vi "sub vi - calibration v2.vi"(6 "Samples":dbl, 8 "Task2":dbl, 9 "Task1":dbl, 10 "Task0":dbl, 11 "Temp Test Cal":dbl) -> ()   [LabVIEW 2017]
panel:
  out "UPDATE":bool
  in  "stop":bool
  in  "Tab Control":T1(tab)
  out "1-2(TN) Run":dbl
  out "1-2(TL) Run":dbl
  out "1-1(TN) Run":dbl
  out "1-1(TL) Run":dbl
  out "LAB01-1 (GRAPH)":dynamicdata(graph)
  out "LAB01-2 (GRAPH)":dynamicdata(graph)
  in  "LAB01 (CAL)":T2 {"2 (TN) cal" min=0.0 step=0.01 format="%.2f"; "2 (TL) cal" min=0.0 step=0.01 format="%.2f"; "2 (PF) cal" min=0.0 step=0.01 format="%.2f"; "2 (V) cal" min=0.0 step=0.01 format="%.2f"; "2 (A) cal" min=0.0 step=0.01 format="%.2f"; "1 (TN) cal" min=0.0 step=0.01 format="%.2f"; "1 (TL) cal" min=0.0 step=0.01 format="%.2f"; "1 (PF) cal" min=0.0 step=0.01 format="%.2f"; "1 (V) cal" min=0.0 step=0.01 format="%.2f"; "1  (A) cal" min=0.0 step=0.01 format="%.2f"}
  out "LAB01 (SIGNALS)":T3 {"2 (PF)" format="%.2f"; "2 (A)" format="%.1f"; "1 (PF)" format="%.2f"; "1 (A)" format="%.1f"}
  out "2-2(TN) Run":dbl
  out "2-2(TL) Run":dbl
  out "2-1(TN) Run":dbl
  out "2-1(TL) Run":dbl
  out "LAB02 (SIGNALS)":T3 {"2 (PF)" format="%.2f"; "2 (A)" format="%.1f"; "1 (PF)" format="%.2f"; "1 (A)" format="%.1f"}
  in  "LAB02 (CAL)":T4 {"2 (TN) cal" min=0.0 step=0.01 format="%.2f"; "2 (TL) cal" min=0.0 step=0.01 format="%.2f"; "2 (PF) cal" min=0.0 step=0.01 format="%.2f"; "2 (V) cal" min=0.0 step=0.01 format="%.2f"; "2 (A) cal" min=0.0 step=0.01 format="%.2f"; "1 (TN) cal" min=0.0 step=0.01 format="%.2f"; "1 (TL) cal" min=0.0 step=0.01 format="%.2f"; "1 (PF) cal" min=0.0 step=0.01 format="%.2f"; "1 (V) cal" min=0.0 step=0.01 format="%.2f"; "1 (A) cal" min=0.0 step=0.01 format="%.2f"}
  out "LAB02-2 (GRAPH)":dynamicdata(graph)
  out "LAB02-1 (GRAPH)":dynamicdata(graph)
  out "3-2(TN) Run":dbl
  out "3-2(TL) Run":dbl
  out "3-1(TN) Run":dbl
  out "3-1(TL) Run":dbl
  out "LAB03 (SIGNALS)":T3 {"2 (PF)" format="%.2f"; "2 (A)" format="%.1f"; "1 (PF)" format="%.2f"; "1 (A)" format="%.1f"}
  in  "LAB03 (CAL)":T2 {"2 (TN) cal" min=0.0 step=0.01 format="%.2f"; "2 (TL) cal" min=0.0 step=0.01 format="%.2f"; "2 (PF) cal" min=0.0 step=0.01 format="%.2f"; "2 (V) cal" min=0.0 step=0.01 format="%.2f"; "2 (A) cal" min=0.0 step=0.01 format="%.2f"; "1 (TN) cal" min=0.0 step=0.01 format="%.2f"; "1 (TL) cal" min=0.0 step=0.01 format="%.2f"; "1 (PF) cal" min=0.0 step=0.01 format="%.2f"; "1 (V) cal" min=0.0 step=0.01 format="%.2f"; "1  (A) cal" min=0.0 step=0.01 format="%.2f"}
  out "LAB03-2 (GRAPH)":dynamicdata(graph)
  out "LAB03-1 (GRAPH)":dynamicdata(graph)
  out "4-2(TN) Run":dbl
  out "4-2(TL) Run":dbl
  out "4-1(TN) Run":dbl
  out "4-1(TL) Run":dbl
  out "LAB04 (SIGNALS)":T3 {"2 (PF)" format="%.2f"; "2 (A)" format="%.1f"; "1 (PF)" format="%.2f"; "1 (A)" format="%.1f"}
  in  "LAB04 (CAL)":T2 {"2 (TN) cal" min=0.0 step=0.01 format="%.2f"; "2 (TL) cal" min=0.0 step=0.01 format="%.2f"; "2 (PF) cal" min=0.0 step=0.01 format="%.2f"; "2 (V) cal" min=0.0 step=0.01 format="%.2f"; "2 (A) cal" min=0.0 step=0.01 format="%.2f"; "1 (TN) cal" min=0.0 step=0.01 format="%.2f"; "1 (TL) cal" min=0.0 step=0.01 format="%.2f"; "1 (PF) cal" min=0.0 step=0.01 format="%.2f"; "1 (V) cal" min=0.0 step=0.01 format="%.2f"; "1  (A) cal" min=0.0 step=0.01 format="%.2f"}
  out "LAB04-2 (GRAPH)":dynamicdata(graph)
  out "LAB04-1 (GRAPH)":dynamicdata(graph)
  in  "LAB05 (CAL) 2":T5 {"2  (A)Zero Offset 1" min=0.0 step=0.01 format="%.2f"; "1  (A)Zero Offset" min=0.0 step=0.01 format="%.2f"; "2 (TN) cal" min=0.0 step=0.01 format="%.2f"; "2 (TL) cal" min=0.0 step=0.01 format="%.2f"; "2 (PF) cal" min=0.0 step=0.01 format="%.2f"; "2 (V) cal" min=0.0 step=0.01 format="%.2f"; "2 (A) cal" min=0.0 step=0.01 format="%.2f"; "1 (TN) cal" min=0.0 step=0.01 format="%.2f"; "1 (TL) cal" min=0.0 step=0.01 format="%.2f"; "1 (PF) cal" min=0.0 step=0.01 format="%.2f"; "1 (V) cal" min=0.0 step=0.01 format="%.2f"; "1  (A) cal" min=0.0 step=0.01 format="%.2f"}
  out "5-2(TN) Run":dbl
  out "5-2(TL) Run":dbl
  out "5-1(TN) Run":dbl
  out "5-1(TL) Run":dbl
  out "LAB05 (SIGNALS)":T3 {"2 (PF)" format="%.2f"; "2 (A)" format="%.1f"; "1 (PF)" format="%.2f"; "1 (A)" format="%.1f"}
  out "LAB05-2 (GRAPH)":dynamicdata(graph)
  out "LAB05-1 (GRAPH)":dynamicdata(graph)
  in  "TEMP REF cal":dbl
  out "AMBIENT TEMP REF":dbl format="%.1f"
  out "Data2":waveform(dbl)[](graph)
  out "Data1":waveform(dbl)[](graph)
  out "Data0":waveform(dbl)[](graph)
  out "Analog Loop Time":dbl
  out "Temperature data error":bool
  out "file error out":errorcluster
  out "AI Error":errorcluster[](array[cluster])
  out "data 0":waveform(dbl)[](array[waveform])
  out "data 1":waveform(dbl)[](array[waveform])
  out "data 2":waveform(dbl)[](array[waveform])
  # "This value is only applied during\ntesting to adjust for insulatred probe\nprofile during current flow temp rise.\nIf any change is made here, make sure\nvalue is changed to same value on\nADM tab."
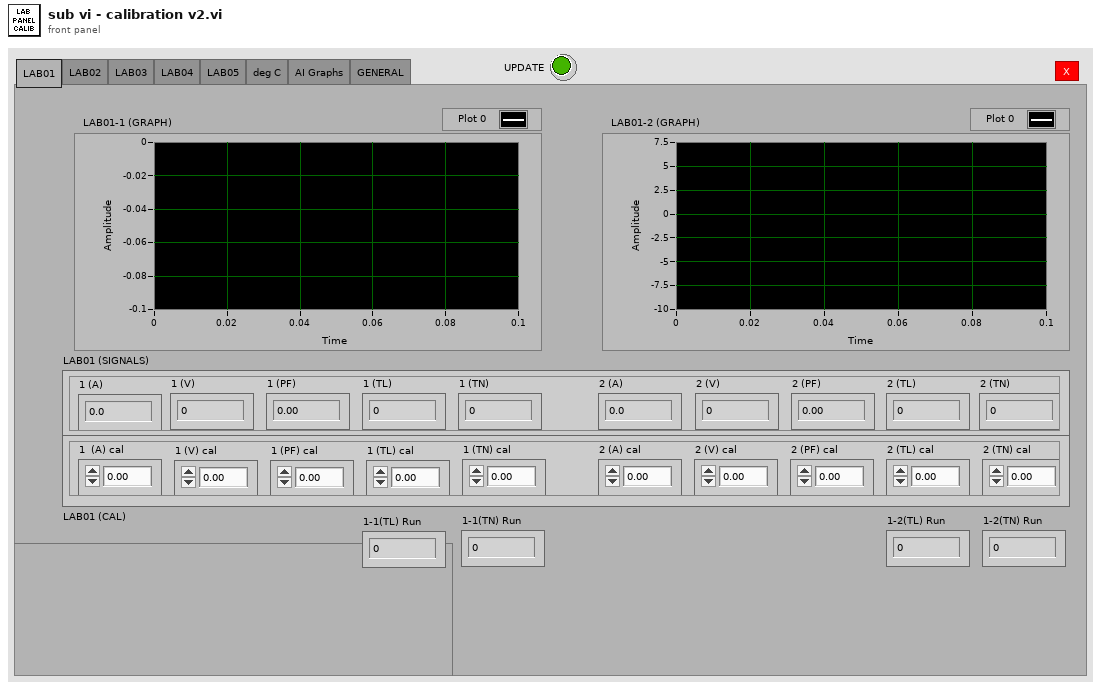
[diagram p1: front panel]
types:
  T1 = enum32{"LAB01", "LAB02", "LAB03", "LAB04", "LAB05", "deg C", "AI Graphs", "GENERAL"}
  T2 = cluster{"1  (A) cal":dbl, "1 (V) cal":dbl, "1 (PF) cal":dbl, "1 (TL) cal":dbl, "1 (TN) cal":dbl, "2 (A) cal":dbl, "2 (V) cal":dbl, "2 (PF) cal":dbl, "2 (TL) cal":dbl, "2 (TN) cal":dbl}
  T3 = cluster{"1 (TL)":dbl, "1 (TN)":dbl, "2 (TL)":dbl, "2 (TN)":dbl, "1 (A)":dbl, "1 (V)":dbl, "1 (PF)":dbl, "2 (A)":dbl, "2 (V)":dbl, "2 (PF)":dbl}
  T4 = cluster{"1 (A) cal":dbl, "1 (V) cal":dbl, "1 (PF) cal":dbl, "1 (TL) cal":dbl, "1 (TN) cal":dbl, "2 (A) cal":dbl, "2 (V) cal":dbl, "2 (PF) cal":dbl, "2 (TL) cal":dbl, "2 (TN) cal":dbl}
  T5 = cluster{"1  (A) cal":dbl, "1 (V) cal":dbl, "1 (PF) cal":dbl, "1 (TL) cal":dbl, "1 (TN) cal":dbl, "2 (A) cal":dbl, "2 (V) cal":dbl, "2 (PF) cal":dbl, "2 (TL) cal":dbl, "2 (TN) cal":dbl, "1  (A)Zero Offset":dbl, "2  (A)Zero Offset 1":dbl}
  T6 = enum16{"open", "replace", "create", "open or create", "replace or create", "replace or create with confirmation"}
  T7 = cluster{"LAB01-1 (A)":dbl, "LAB01-1 (V)":dbl, "LAB01-1 (PF)":dbl, "LAB01-2 (A)":dbl, "LAB01-2 (V)":dbl, "LAB01-2 (PF)":dbl}
  T8 = cluster{"LAB02-1 (A)":dbl, "LAB02-1 (V)":dbl, "LAB02-1 (PF)":dbl, "LAB02-2 (A)":dbl, "LAB02-2 (V)":dbl, "LAB02-2 (PF)":dbl}
  T9 = cluster{"LAB03-1 (A)":dbl, "LAB03-1 (V)":dbl, "LAB03-1 (PF)":dbl, "LAB03-2 (A)":dbl, "LAB03-2 (V)":dbl, "LAB03-2 (PF)":dbl}
  T10 = cluster{"LAB04-1 (A)":dbl, "LAB04-1 (V)":dbl, "LAB04-1 (PF)":dbl, "LAB04-2 (A)":dbl, "LAB04-2 (V)":dbl, "LAB04-2 (PF)":dbl}
  T11 = cluster{"LAB05-1 (A)":dbl, "LAB05-1 (V)":dbl, "LAB05-1 (PF)":dbl, "LAB05-2 (A)":dbl, "LAB05-2 (V)":dbl, "LAB05-2 (PF)":dbl}
  T12 = cluster{"T1":dbl, "T2":dbl, "T3":dbl, "T4":dbl, "ID":dbl, "ER":dbl}
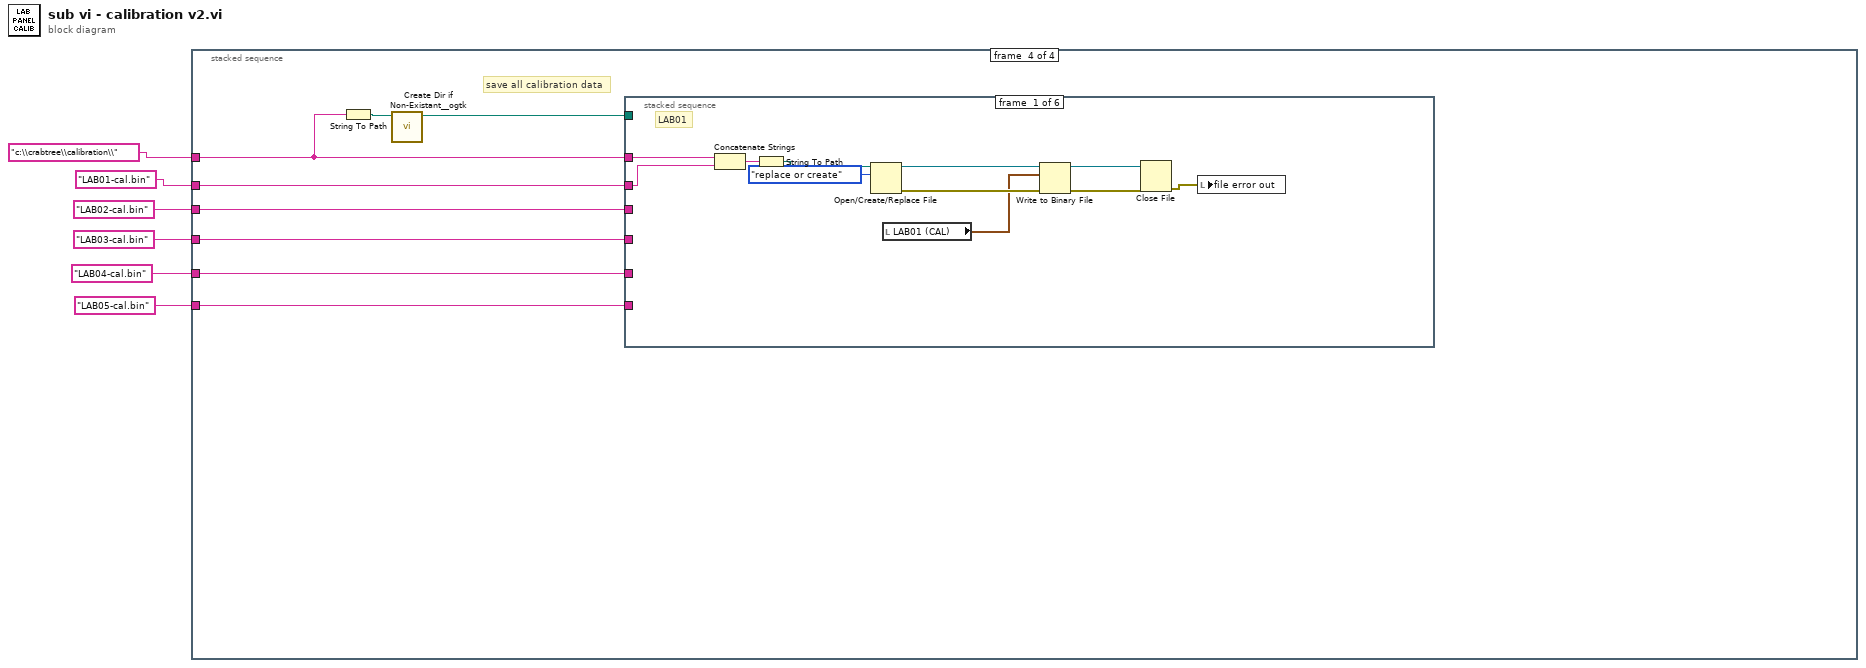
[diagram p0: block diagram]
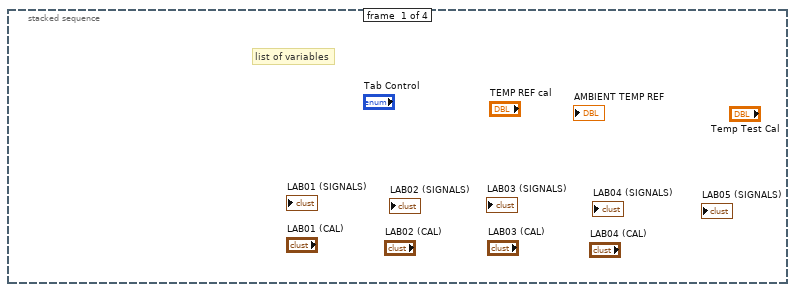
[diagram p2: hidden frame]
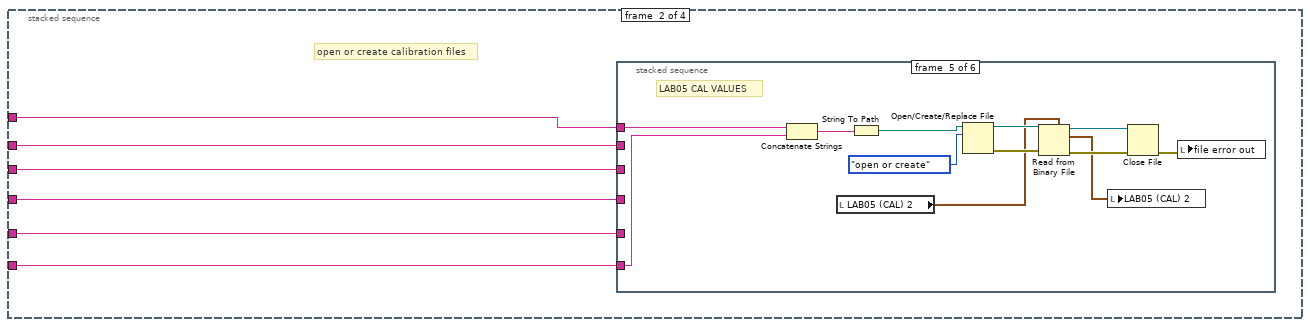
[diagram p3: hidden frame]
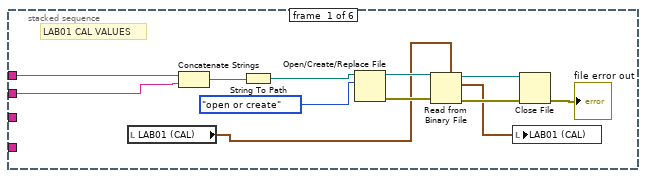
[diagram p4: hidden frame]
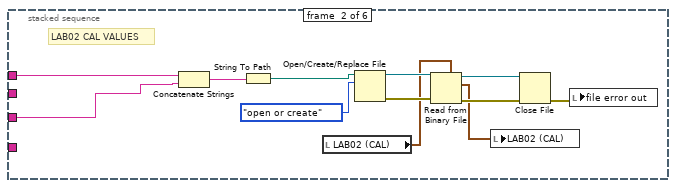
[diagram p5: hidden frame]
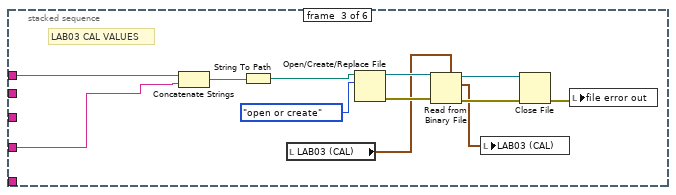
[diagram p6: hidden frame]
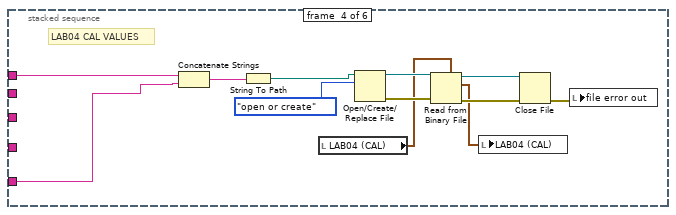
[diagram p7: hidden frame]
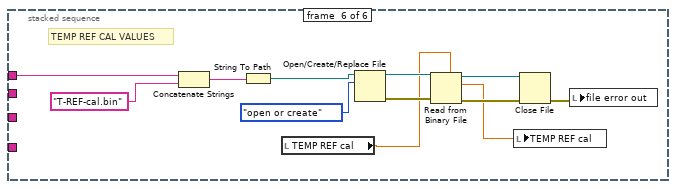
[diagram p8: hidden frame]
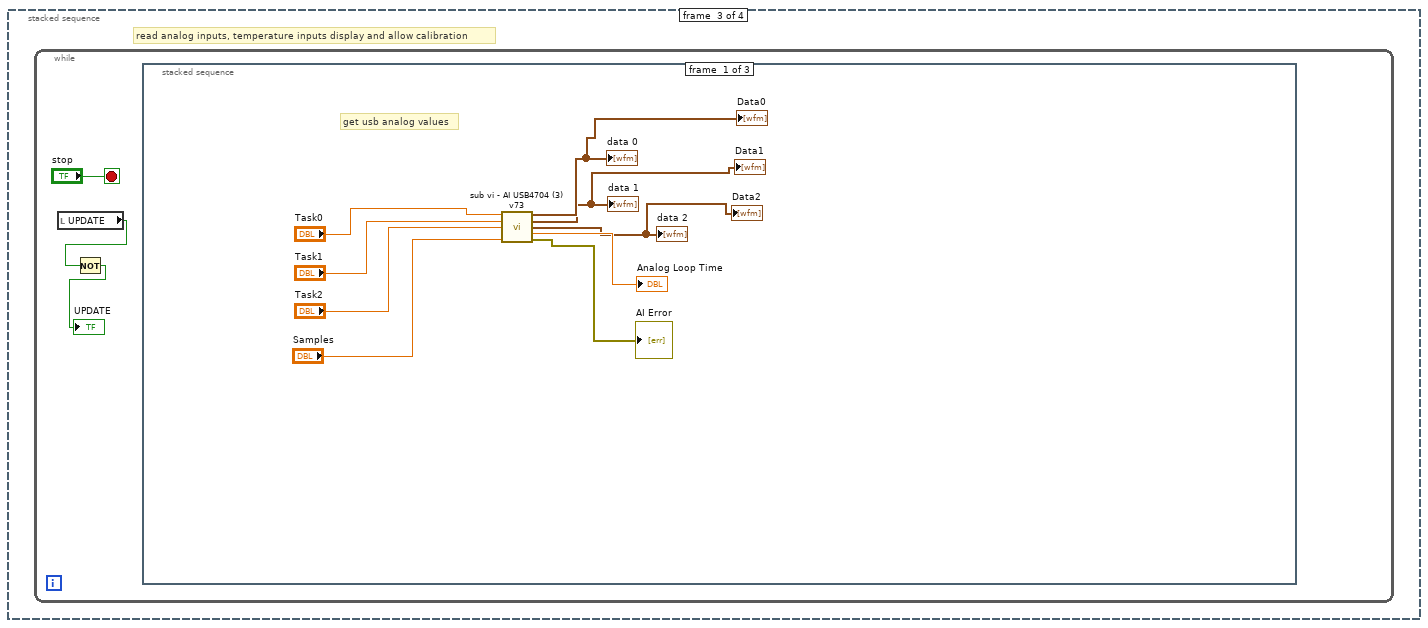
[diagram p9: hidden frame]
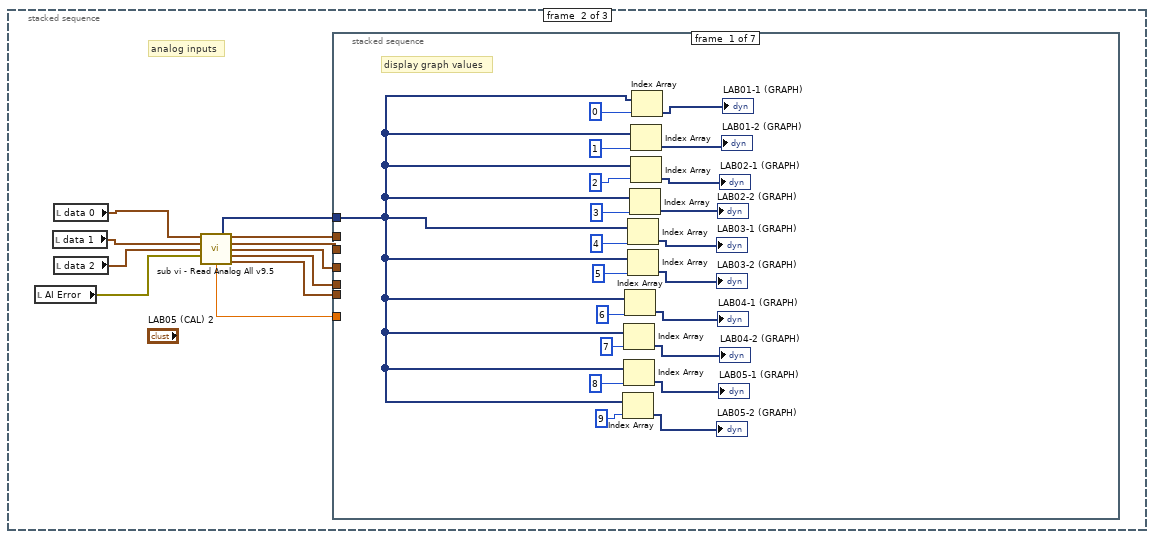
[diagram p10: hidden frame]
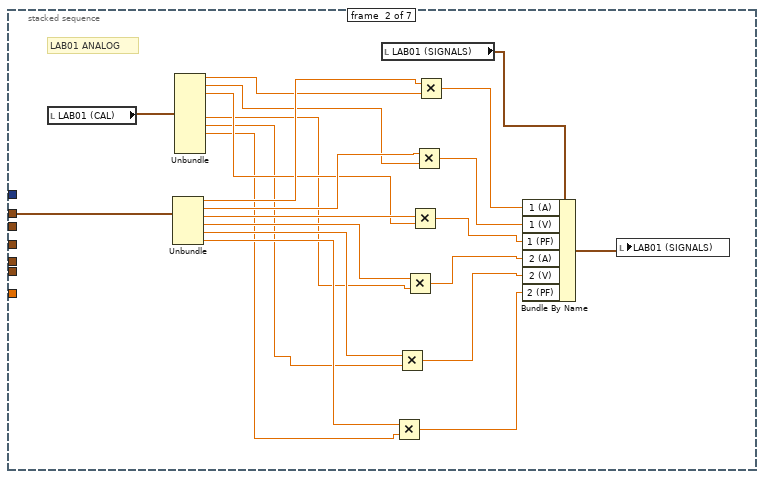
[diagram p11: hidden frame]
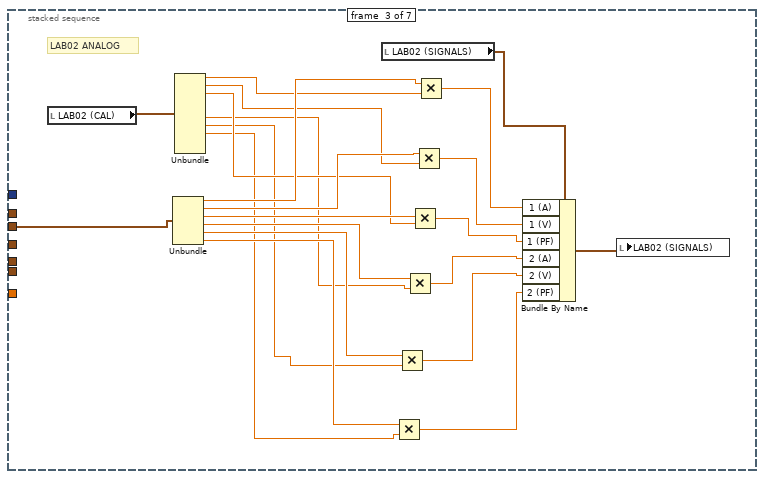
[diagram p12: hidden frame]
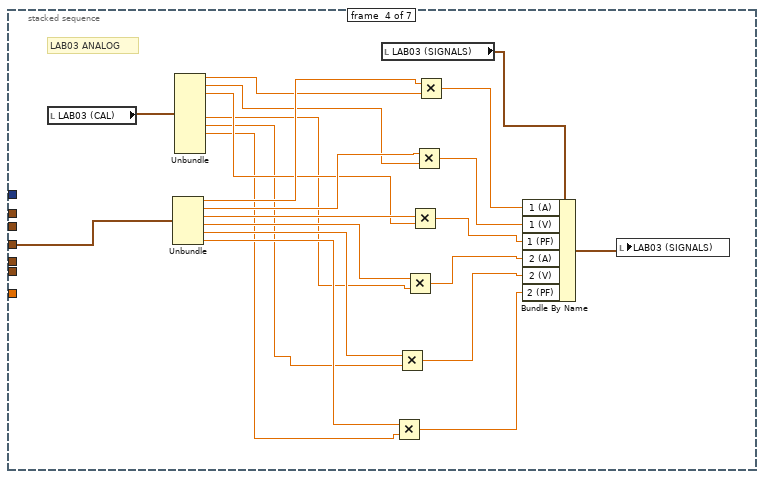
[diagram p13: hidden frame]
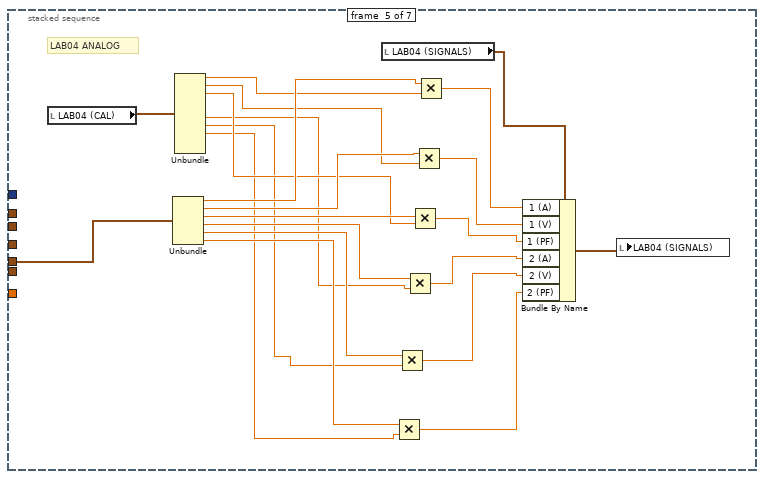
[diagram p14: hidden frame]
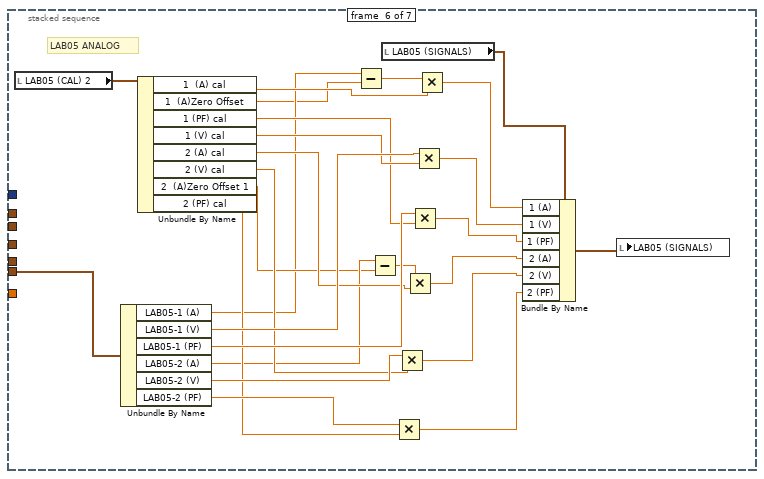
[diagram p15: hidden frame]
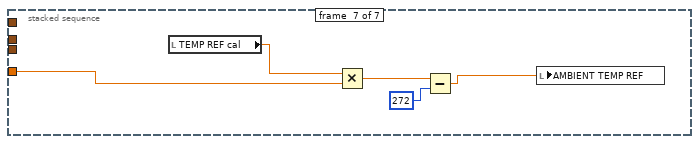
[diagram p16: hidden frame]
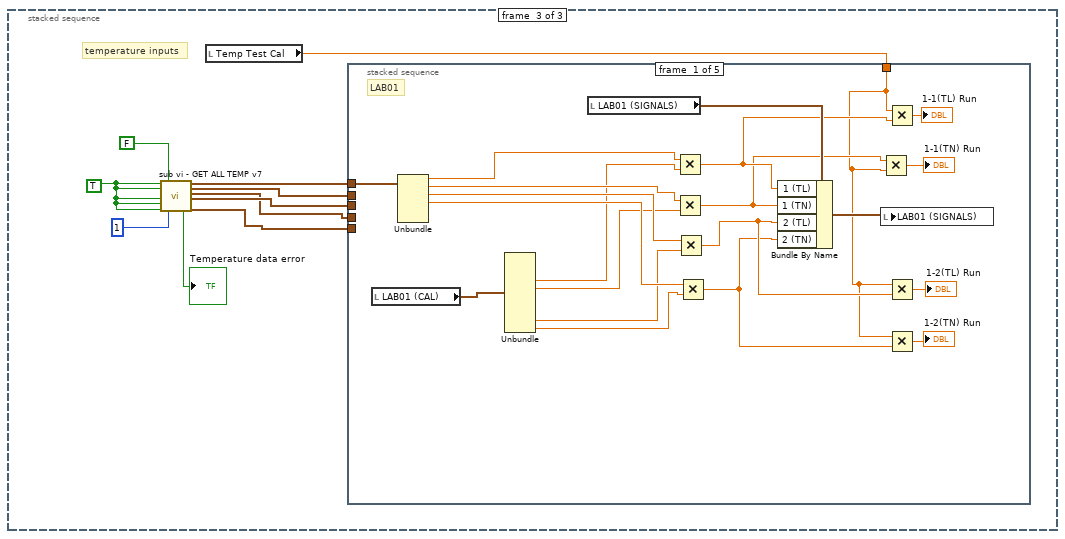
[diagram p17: hidden frame]
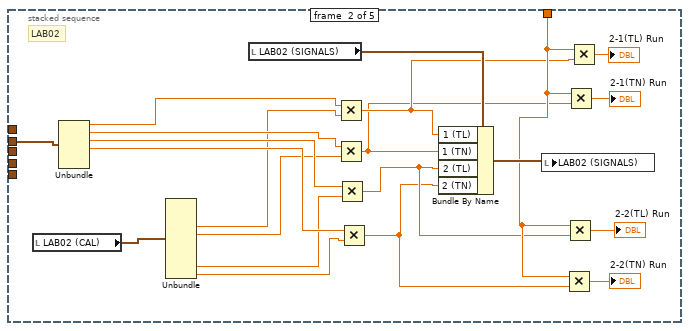
[diagram p18: hidden frame]
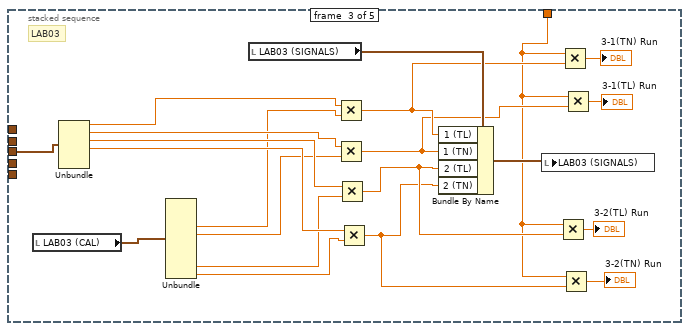
[diagram p19: hidden frame]
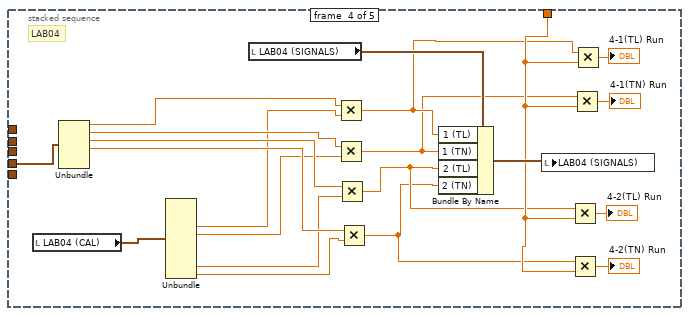
[diagram p20: hidden frame]
diagram:
  n1 = stacked-sequence {
    tunnel: "c:\\crabtree\\calibration\\" -> [_ w12 _ w365]
    tunnel: "LAB01-cal.bin" -> [_ w11 _ w370]
    tunnel: "LAB02-cal.bin" -> [_ w10 _ w369]
    tunnel: "LAB03-cal.bin" -> [_ w9 _ w368]
    tunnel: "LAB04-cal.bin" -> [_ w8 _ w367]
    tunnel: "LAB05-cal.bin" -> [_ w7 _ w366]
    frame #0 {
      # "list of variables"
    }
    frame #1 {
      # "open or create calibration files"
      n2 = stacked-sequence {
        tunnel: w12 -> [w24 w36 w48 w60 w72 w84]
        tunnel: w11 -> [w15 _ _ _ _ _]
        tunnel: w10 -> [_ w27 _ _ _ _]
        tunnel: w9 -> [_ _ w39 _ _ _]
        tunnel: w8 -> [_ _ _ w52 _ _]
        tunnel: w7 -> [_ _ _ _ w63 _]
        frame #0 {
          # "LAB01 CAL VALUES"
          n3 = local read "LAB01 (CAL)"() -> (w14:T2)
          n4 = Concatenate Strings(w24, w15) -> (w23:string)
          n5 = String To Path(string=w23) -> (path=w22:path)
          n6 = Open/Create/Replace File(file path (use dialog)=w22, operation (0:open)=T6."open or create") -> (refnum out=w21:refnum<file>, error out=w20:errorcluster)  [unwired: 4 in, 1 out]
          n7 = Read from Binary File(5:w14, 8:w20, 11:w21) -> (0:w18:errorcluster, 2:w13:T2, 3:w19:refnum<file>)  [unwired: 3 in, 1 out]
          n8 = local write "LAB01 (CAL)"(w13) -> ()
          n9 = Close File(refnum=w19, error in=w18) -> (error out=→"file error out":errorcluster)  [unwired: 1 out]
        }
        frame #1 {
          # "LAB02 CAL VALUES"
          n10 = Concatenate Strings(w36, w27) -> (w35:string)
          n11 = String To Path(string=w35) -> (path=w34:path)
          n12 = local read "LAB02 (CAL)"() -> (w26:T4)
          n13 = Open/Create/Replace File(file path (use dialog)=w34, operation (0:open)=T6."open or create") -> (refnum out=w33:refnum<file>, error out=w32:errorcluster)  [unwired: 4 in, 1 out]
          n14 = Read from Binary File(5:w26, 8:w32, 11:w33) -> (0:w30:errorcluster, 2:w25:T4, 3:w31:refnum<file>)  [unwired: 3 in, 1 out]
          n15 = local write "LAB02 (CAL)"(w25) -> ()
          n16 = Close File(refnum=w31, error in=w30) -> (error out=w28:errorcluster)  [unwired: 1 out]
          n17 = local write "file error out"(w28) -> ()
        }
        frame #2 {
          # "LAB03 CAL VALUES"
          n18 = Concatenate Strings(w48, w39) -> (w47:string)
          n19 = String To Path(string=w47) -> (path=w46:path)
          n20 = local read "LAB03 (CAL)"() -> (w38:T2)
          n21 = Open/Create/Replace File(file path (use dialog)=w46, operation (0:open)=T6."open or create") -> (refnum out=w45:refnum<file>, error out=w44:errorcluster)  [unwired: 4 in, 1 out]
          n22 = Read from Binary File(5:w38, 8:w44, 11:w45) -> (0:w42:errorcluster, 2:w37:T2, 3:w43:refnum<file>)  [unwired: 3 in, 1 out]
          n23 = local write "LAB03 (CAL)"(w37) -> ()
          n24 = Close File(refnum=w43, error in=w42) -> (error out=w40:errorcluster)  [unwired: 1 out]
          n25 = local write "file error out"(w40) -> ()
        }
        frame #3 {
          # "LAB04 CAL VALUES"
          n26 = Concatenate Strings(w60, w52) -> (w59:string)
          n27 = String To Path(string=w59) -> (path=w58:path)
          n28 = local read "LAB04 (CAL)"() -> (w50:T2)
          n29 = Open/Create/Replace File(file path (use dialog)=w58, operation (0:open)=T6."open or create") -> (refnum out=w57:refnum<file>, error out=w56:errorcluster)  [unwired: 4 in, 1 out]
          n30 = Read from Binary File(5:w50, 8:w56, 11:w57) -> (0:w54:errorcluster, 2:w49:T2, 3:w55:refnum<file>)  [unwired: 3 in, 1 out]
          n31 = local write "LAB04 (CAL)"(w49) -> ()
          n32 = Close File(refnum=w55, error in=w54) -> (error out=w53:errorcluster)  [unwired: 1 out]
          n33 = local write "file error out"(w53) -> ()
        }
        frame #4 {
          # "LAB05 CAL VALUES"
          n34 = Concatenate Strings(w72, w63) -> (w71:string)
          n35 = local read "LAB05 (CAL) 2"() -> (w62:T5)
          n36 = String To Path(string=w71) -> (path=w70:path)
          n37 = Open/Create/Replace File(file path (use dialog)=w70, operation (0:open)=T6."open or create") -> (refnum out=w69:refnum<file>, error out=w68:errorcluster)  [unwired: 4 in, 1 out]
          n38 = Read from Binary File(5:w62, 8:w68, 11:w69) -> (0:w66:errorcluster, 2:w61:T5, 3:w67:refnum<file>)  [unwired: 3 in, 1 out]
          n39 = local write "LAB05 (CAL) 2"(w61) -> ()
          n40 = Close File(refnum=w67, error in=w66) -> (error out=w64:errorcluster)  [unwired: 1 out]
          n41 = local write "file error out"(w64) -> ()
        }
        frame #5 {
          # "TEMP REF CAL VALUES"
          n42 = Concatenate Strings(w84, "T-REF-cal.bin") -> (w83:string)
          n43 = String To Path(string=w83) -> (path=w82:path)
          n44 = local read "TEMP REF cal"() -> (w74:dbl)
          n45 = Open/Create/Replace File(file path (use dialog)=w82, operation (0:open)=T6."open or create") -> (refnum out=w81:refnum<file>, error out=w80:errorcluster)  [unwired: 4 in, 1 out]
          n46 = Read from Binary File(5:w74, 8:w80, 11:w81) -> (0:w78:errorcluster, 2:w73:dbl, 3:w79:refnum<file>)  [unwired: 3 in, 1 out]
          n47 = local write "TEMP REF cal"(w73) -> ()
          n48 = Close File(refnum=w79, error in=w78) -> (error out=w76:errorcluster)  [unwired: 1 out]
          n49 = local write "file error out"(w76) -> ()
        }
      }
    }
    frame #2 {
      # "read analog inputs, temperature inputs display and allow calibration"
      n50 = while {
        stop <- "stop" stop-if-true
        n51 = local read "UPDATE"() -> (w85:bool)
        n52 = Not(x=w85) -> (.not. x?=→"UPDATE":bool)
        n53 = stacked-sequence {
          frame #0 {
            # "get usb analog values"
            n54 = call "sub vi - AI USB4704 (3) v73.vi"("Task0"="Task0", "Task1"="Task1", "Task2"="Task2", "SAMPLES"="Samples") -> ("data 0"=→"data 0" →"Data0":waveform(dbl)[], "data 1"=→"data 1" →"Data1":waveform(dbl)[], "data 2"=→"data 2" →"Data2":waveform(dbl)[], "loop time"=→"Analog Loop Time":dbl, "error array"=→"AI Error":errorcluster[])  [unwired: 5 in, 2 out]
          }
          frame #1 {
            # "analog inputs"
            n55 = local read "AI Error"() -> (w97:errorcluster[])
            n56 = local read "data 1"() -> (w99:waveform(dbl)[])
            n57 = local read "data 0"() -> (w100:waveform(dbl)[])
            n58 = local read "data 2"() -> (w98:waveform(dbl)[])
            n59 = call "sub vi - Read Analog All v9.5.vi"("data 0"=w100, "data 1"=w99, "data 2"=w98, "AI Error"=w97) -> ("array GRAPH"=w107:dynamicdata[], "LAB01"=w106:T7, "LAB02"=w105:T8, "LAB03"=w104:T9, "LAB04"=w103:T10, "deg C"=w101:dbl, "LAB05"=w102:T11)  [unwired: 3 in, 2 out]
            n60 = stacked-sequence {
              tunnel: w107 -> [w127 _ _ _ _ _ _]
              tunnel: w106 -> [_ w149 _ _ _ _ _]
              tunnel: w104 -> [_ _ _ w173 _ _ _]
              tunnel: w105 -> [_ _ w151 _ _ _ _]
              tunnel: w103 -> [_ _ _ _ w195 _ _]
              tunnel: w102 -> [_ _ _ _ _ w228 _]
              tunnel: w101 -> [_ _ _ _ _ _ w246]
              frame #0 {
                # "display graph values"
                n61 = Index Array(array=w127, index=9) -> (element=→"LAB05-2 (GRAPH)":dynamicdata)
                n62 = Index Array(array=w127, index=7) -> (element=→"LAB04-2 (GRAPH)":dynamicdata)
                n63 = Index Array(array=w127, index=8) -> (element=→"LAB05-1 (GRAPH)":dynamicdata)
                n64 = Index Array(array=w127, index=6) -> (element=→"LAB04-1 (GRAPH)":dynamicdata)
                n65 = Index Array(array=w127, index=4) -> (element=→"LAB03-1 (GRAPH)":dynamicdata)
                n66 = Index Array(array=w127, index=5) -> (element=→"LAB03-2 (GRAPH)":dynamicdata)
                n67 = Index Array(array=w127, index=3) -> (element=→"LAB02-2 (GRAPH)":dynamicdata)
                n68 = Index Array(array=w127, index=1) -> (element=→"LAB01-2 (GRAPH)":dynamicdata)
                n69 = Index Array(array=w127, index=2) -> (element=→"LAB02-1 (GRAPH)":dynamicdata)
                n70 = Index Array(array=w127, index=0) -> (element=→"LAB01-1 (GRAPH)":dynamicdata)
              }
              frame #1 {
                # "LAB01 ANALOG"
                n71 = local read "LAB01 (CAL)"() -> (w150:T2)
                n72 = Unbundle(w149) -> ("LAB01-1 (A)"=w148:dbl, "LAB01-1 (V)"=w147:dbl, "LAB01-1 (PF)"=w146:dbl, "LAB01-2 (A)"=w145:dbl, "LAB01-2 (V)"=w144:dbl, "LAB01-2 (PF)"=w143:dbl)
                n73 = Unbundle(w150) -> ("1  (A) cal"=w142:dbl, "1 (V) cal"=w141:dbl, "1 (PF) cal"=w140:dbl, "2 (A) cal"=w139:dbl, "2 (V) cal"=w138:dbl, "2 (PF) cal"=w137:dbl)  [unwired: 4 out]
                n74 = local read "LAB01 (SIGNALS)"() -> (w136:T3)
                n75 = Multiply(x=w143, y=w137) -> (x*y=w130:dbl)
                n76 = Multiply(x=w144, y=w138) -> (x*y=w131:dbl)
                n77 = Multiply(x=w145, y=w139) -> (x*y=w132:dbl)
                n78 = Multiply(x=w146, y=w140) -> (x*y=w133:dbl)
                n79 = Multiply(x=w147, y=w141) -> (x*y=w134:dbl)
                n80 = Multiply(x=w148, y=w142) -> (x*y=w135:dbl)
                n81 = Bundle By Name(cluster=w136, "1 (A)"=w135, "1 (V)"=w134, "1 (PF)"=w133, "2 (A)"=w132, "2 (V)"=w131, "2 (PF)"=w130) -> (w129:T3)
                n82 = local write "LAB01 (SIGNALS)"(w129) -> ()
              }
              frame #2 {
                # "LAB02 ANALOG"
                n83 = local read "LAB02 (CAL)"() -> (w172:T4)
                n84 = Unbundle(w151) -> ("LAB02-1 (A)"=w171:dbl, "LAB02-1 (V)"=w170:dbl, "LAB02-1 (PF)"=w169:dbl, "LAB02-2 (A)"=w168:dbl, "LAB02-2 (V)"=w167:dbl, "LAB02-2 (PF)"=w166:dbl)
                n85 = Unbundle(w172) -> ("1 (A) cal"=w165:dbl, "1 (V) cal"=w164:dbl, "1 (PF) cal"=w163:dbl, "2 (A) cal"=w162:dbl, "2 (V) cal"=w161:dbl, "2 (PF) cal"=w160:dbl)  [unwired: 4 out]
                n86 = local read "LAB02 (SIGNALS)"() -> (w159:T3)
                n87 = Multiply(x=w166, y=w160) -> (x*y=w153:dbl)
                n88 = Multiply(x=w167, y=w161) -> (x*y=w154:dbl)
                n89 = Multiply(x=w168, y=w162) -> (x*y=w155:dbl)
                n90 = Multiply(x=w169, y=w163) -> (x*y=w156:dbl)
                n91 = Multiply(x=w170, y=w164) -> (x*y=w157:dbl)
                n92 = Multiply(x=w171, y=w165) -> (x*y=w158:dbl)
                n93 = Bundle By Name(cluster=w159, "1 (A)"=w158, "1 (V)"=w157, "1 (PF)"=w156, "2 (A)"=w155, "2 (V)"=w154, "2 (PF)"=w153) -> (w152:T3)
                n94 = local write "LAB02 (SIGNALS)"(w152) -> ()
              }
              frame #3 {
                # "LAB03 ANALOG"
                n95 = local read "LAB03 (CAL)"() -> (w194:T2)
                n96 = Unbundle(w173) -> ("LAB03-1 (A)"=w193:dbl, "LAB03-1 (V)"=w192:dbl, "LAB03-1 (PF)"=w191:dbl, "LAB03-2 (A)"=w190:dbl, "LAB03-2 (V)"=w189:dbl, "LAB03-2 (PF)"=w188:dbl)
                n97 = Unbundle(w194) -> ("1  (A) cal"=w187:dbl, "1 (V) cal"=w186:dbl, "1 (PF) cal"=w185:dbl, "2 (A) cal"=w184:dbl, "2 (V) cal"=w183:dbl, "2 (PF) cal"=w182:dbl)  [unwired: 4 out]
                n98 = local read "LAB03 (SIGNALS)"() -> (w181:T3)
                n99 = Multiply(x=w188, y=w182) -> (x*y=w175:dbl)
                n100 = Multiply(x=w189, y=w183) -> (x*y=w176:dbl)
                n101 = Multiply(x=w190, y=w184) -> (x*y=w177:dbl)
                n102 = Multiply(x=w191, y=w185) -> (x*y=w178:dbl)
                n103 = Multiply(x=w192, y=w186) -> (x*y=w179:dbl)
                n104 = Multiply(x=w193, y=w187) -> (x*y=w180:dbl)
                n105 = Bundle By Name(cluster=w181, "1 (A)"=w180, "1 (V)"=w179, "1 (PF)"=w178, "2 (A)"=w177, "2 (V)"=w176, "2 (PF)"=w175) -> (w174:T3)
                n106 = local write "LAB03 (SIGNALS)"(w174) -> ()
              }
              frame #4 {
                # "LAB04 ANALOG"
                n107 = local read "LAB04 (CAL)"() -> (w216:T2)
                n108 = Unbundle(w195) -> ("LAB04-1 (A)"=w215:dbl, "LAB04-1 (V)"=w214:dbl, "LAB04-1 (PF)"=w213:dbl, "LAB04-2 (A)"=w212:dbl, "LAB04-2 (V)"=w211:dbl, "LAB04-2 (PF)"=w210:dbl)
                n109 = Unbundle(w216) -> ("1  (A) cal"=w209:dbl, "1 (V) cal"=w208:dbl, "1 (PF) cal"=w207:dbl, "2 (A) cal"=w206:dbl, "2 (V) cal"=w205:dbl, "2 (PF) cal"=w204:dbl)  [unwired: 4 out]
                n110 = local read "LAB04 (SIGNALS)"() -> (w203:T3)
                n111 = Multiply(x=w210, y=w204) -> (x*y=w197:dbl)
                n112 = Multiply(x=w211, y=w205) -> (x*y=w198:dbl)
                n113 = Multiply(x=w212, y=w206) -> (x*y=w199:dbl)
                n114 = Multiply(x=w213, y=w207) -> (x*y=w200:dbl)
                n115 = Multiply(x=w214, y=w208) -> (x*y=w201:dbl)
                n116 = Multiply(x=w215, y=w209) -> (x*y=w202:dbl)
                n117 = Bundle By Name(cluster=w203, "1 (A)"=w202, "1 (V)"=w201, "1 (PF)"=w200, "2 (A)"=w199, "2 (V)"=w198, "2 (PF)"=w197) -> (w196:T3)
                n118 = local write "LAB04 (SIGNALS)"(w196) -> ()
              }
              frame #5 {
                # "LAB05 ANALOG"
                n119 = local read "LAB05 (CAL) 2"() -> (w227:T5)
                n120 = Unbundle By Name(w228) -> ("LAB05-1 (A)"=w219:dbl, "LAB05-1 (V)"=w242:dbl, "LAB05-1 (PF)"=w241:dbl, "LAB05-2 (A)"=w223:dbl, "LAB05-2 (V)"=w240:dbl, "LAB05-2 (PF)"=w239:dbl)
                n121 = Unbundle By Name(w227) -> ("1  (A) cal"=w220:dbl, "1  (A)Zero Offset"=w218:dbl, "1 (PF) cal"=w225:dbl, "1 (V) cal"=w226:dbl, "2 (A) cal"=w238:dbl, "2 (V) cal"=w237:dbl, "2  (A)Zero Offset 1"=w222:dbl, "2 (PF) cal"=w224:dbl)
                n122 = Subtract(x=w219, y=w218) -> (x-y=w217:dbl)
                n123 = Subtract(x=w223, y=w222) -> (x-y=w221:dbl)
                n124 = local read "LAB05 (SIGNALS)"() -> (w236:T3)
                n125 = Multiply(x=w239, y=w224) -> (x*y=w230:dbl)
                n126 = Multiply(x=w240, y=w237) -> (x*y=w231:dbl)
                n127 = Multiply(x=w221, y=w238) -> (x*y=w232:dbl)
                n128 = Multiply(x=w241, y=w225) -> (x*y=w233:dbl)
                n129 = Multiply(x=w242, y=w226) -> (x*y=w234:dbl)
                n130 = Multiply(x=w217, y=w220) -> (x*y=w235:dbl)
                n131 = Bundle By Name(cluster=w236, "1 (A)"=w235, "1 (V)"=w234, "1 (PF)"=w233, "2 (A)"=w232, "2 (V)"=w231, "2 (PF)"=w230) -> (w229:T3)
                n132 = local write "LAB05 (SIGNALS)"(w229) -> ()
              }
              frame #6 {
                n133 = local read "TEMP REF cal"() -> (w247:dbl)
                n134 = Multiply(x=w247, y=w246) -> (x*y=w245:dbl)
                n135 = Subtract(x=w245, y=272) -> (x-y=w243:dbl)
                n136 = local write "AMBIENT TEMP REF"(w243) -> ()
              }
            }
          }
          frame #2 {
            w257 = TRUE
            # "temperature inputs"
            n137 = call "sub vi - GET ALL TEMP v7.vi"("LA01-EN"=w257, "LA02-EN"=w257, "LA03-EN"=w257, "LA04-EN"=w257, "LA05-EN"=w257, "simulate"=FALSE, "Gen Cal Value"=1) -> ("error 1"=→"Temperature data error":bool, "LA01 TEMP"=w255:T12, "LA02 TEMP"=w253:T12, "LA04 TEMP"=w251:T12, "LA03 TEMP"=w252:T12, "LA05 TEMP"=w250:T12)  [unwired: 3 in, 4 out]
            n138 = local read "Temp Test Cal"() -> (w248:dbl)
            n139 = stacked-sequence {
              tunnel: w255 -> [w277 _ _ _ _]
              tunnel: w253 -> [_ w288 _ _ _]
              tunnel: w252 -> [_ _ w309 _ _]
              tunnel: w251 -> [_ _ _ w330 _]
              tunnel: w250 -> [_ _ _ _ w352]
              tunnel: w248 -> [w258 w283 w301 w325 w347]
              frame #0 {
                # "LAB01"
                n140 = local read "LAB01 (CAL)"() -> (w278:T2)
                n141 = Unbundle(w277) -> ("T1"=w276:dbl, "T2"=w275:dbl, "T3"=w274:dbl, "T4"=w273:dbl)  [unwired: 2 out]
                n142 = Unbundle(w278) -> ("1 (TL) cal"=w272:dbl, "1 (TN) cal"=w271:dbl, "2 (TL) cal"=w270:dbl, "2 (TN) cal"=w269:dbl)  [unwired: 6 out]
                n143 = local read "LAB01 (SIGNALS)"() -> (w268:T3)
                n144 = Multiply(x=w276, y=w272) -> (x*y=w265:dbl)
                n145 = Multiply(x=w275, y=w271) -> (x*y=w263:dbl)
                n146 = Multiply(x=w274, y=w270) -> (x*y=w260:dbl)
                n147 = Multiply(x=w273, y=w269) -> (x*y=w259:dbl)
                n148 = Bundle By Name(cluster=w268, "1 (TL)"=w265, "1 (TN)"=w263, "2 (TL)"=w260, "2 (TN)"=w259) -> (w267:T3)
                n149 = Multiply(x=w263, y=w258) -> (x*y=→"1-1(TN) Run":dbl)
                n150 = local write "LAB01 (SIGNALS)"(w267) -> ()
                n151 = Multiply(x=w258, y=w265) -> (x*y=→"1-1(TL) Run":dbl)
                n152 = Multiply(x=w258, y=w260) -> (x*y=→"1-2(TL) Run":dbl)
                n153 = Multiply(x=w258, y=w259) -> (x*y=→"1-2(TN) Run":dbl)
              }
              frame #1 {
                # "LAB02"
                n154 = local read "LAB02 (CAL)"() -> (w299:T4)
                n155 = Unbundle(w288) -> ("T1"=w298:dbl, "T2"=w297:dbl, "T3"=w296:dbl, "T4"=w295:dbl)  [unwired: 2 out]
                n156 = Unbundle(w299) -> ("1 (TL) cal"=w294:dbl, "1 (TN) cal"=w293:dbl, "2 (TL) cal"=w292:dbl, "2 (TN) cal"=w291:dbl)  [unwired: 6 out]
                n157 = local read "LAB02 (SIGNALS)"() -> (w290:T3)
                n158 = Multiply(x=w298, y=w294) -> (x*y=w282:dbl)
                n159 = Multiply(x=w297, y=w293) -> (x*y=w281:dbl)
                n160 = Multiply(x=w296, y=w292) -> (x*y=w280:dbl)
                n161 = Multiply(x=w295, y=w291) -> (x*y=w279:dbl)
                n162 = Bundle By Name(cluster=w290, "1 (TL)"=w282, "1 (TN)"=w281, "2 (TL)"=w280, "2 (TN)"=w279) -> (w289:T3)
                n163 = local write "LAB02 (SIGNALS)"(w289) -> ()
                n164 = Multiply(x=w283, y=w279) -> (x*y=→"2-2(TN) Run":dbl)
                n165 = Multiply(x=w283, y=w280) -> (x*y=→"2-2(TL) Run":dbl)
                n166 = Multiply(x=w283, y=w281) -> (x*y=→"2-1(TN) Run":dbl)
                n167 = Multiply(x=w283, y=w282) -> (x*y=→"2-1(TL) Run":dbl)
              }
              frame #2 {
                # "LAB03"
                n168 = local read "LAB03 (CAL)"() -> (w320:T2)
                n169 = Unbundle(w309) -> ("T1"=w319:dbl, "T2"=w318:dbl, "T3"=w317:dbl, "T4"=w316:dbl)  [unwired: 2 out]
                n170 = Unbundle(w320) -> ("1 (TL) cal"=w315:dbl, "1 (TN) cal"=w314:dbl, "2 (TL) cal"=w313:dbl, "2 (TN) cal"=w312:dbl)  [unwired: 6 out]
                n171 = local read "LAB03 (SIGNALS)"() -> (w311:T3)
                n172 = Multiply(x=w319, y=w315) -> (x*y=w305:dbl)
                n173 = Multiply(x=w318, y=w314) -> (x*y=w304:dbl)
                n174 = Multiply(x=w317, y=w313) -> (x*y=w303:dbl)
                n175 = Multiply(x=w316, y=w312) -> (x*y=w302:dbl)
                n176 = Bundle By Name(cluster=w311, "1 (TL)"=w305, "1 (TN)"=w304, "2 (TL)"=w303, "2 (TN)"=w302) -> (w310:T3)
                n177 = local write "LAB03 (SIGNALS)"(w310) -> ()
                n178 = Multiply(x=w301, y=w303) -> (x*y=→"3-2(TL) Run":dbl)
                n179 = Multiply(x=w301, y=w305) -> (x*y=→"3-1(TN) Run":dbl)
                n180 = Multiply(x=w301, y=w302) -> (x*y=→"3-2(TN) Run":dbl)
                n181 = Multiply(x=w301, y=w304) -> (x*y=→"3-1(TL) Run":dbl)
              }
              frame #3 {
                # "LAB04"
                n182 = local read "LAB04 (CAL)"() -> (w341:T2)
                n183 = Unbundle(w330) -> ("T1"=w340:dbl, "T2"=w339:dbl, "T3"=w338:dbl, "T4"=w337:dbl)  [unwired: 2 out]
                n184 = Unbundle(w341) -> ("1 (TL) cal"=w336:dbl, "1 (TN) cal"=w335:dbl, "2 (TL) cal"=w334:dbl, "2 (TN) cal"=w333:dbl)  [unwired: 6 out]
                n185 = local read "LAB04 (SIGNALS)"() -> (w332:T3)
                n186 = Multiply(x=w340, y=w336) -> (x*y=w324:dbl)
                n187 = Multiply(x=w339, y=w335) -> (x*y=w323:dbl)
                n188 = Multiply(x=w338, y=w334) -> (x*y=w322:dbl)
                n189 = Multiply(x=w337, y=w333) -> (x*y=w321:dbl)
                n190 = Bundle By Name(cluster=w332, "1 (TL)"=w324, "1 (TN)"=w323, "2 (TL)"=w322, "2 (TN)"=w321) -> (w331:T3)
                n191 = local write "LAB04 (SIGNALS)"(w331) -> ()
                n192 = Multiply(x=w322, y=w325) -> (x*y=→"4-2(TL) Run":dbl)
                n193 = Multiply(x=w321, y=w325) -> (x*y=→"4-2(TN) Run":dbl)
                n194 = Multiply(x=w323, y=w325) -> (x*y=→"4-1(TN) Run":dbl)
                n195 = Multiply(x=w324, y=w325) -> (x*y=→"4-1(TL) Run":dbl)
              }
              frame #4 {
                # "LAB05"
                n196 = local read "LAB05 (CAL) 2"() -> (w342:T5)
                n197 = Unbundle(w352) -> ("T1"=w362:dbl, "T2"=w361:dbl, "T3"=w360:dbl, "T4"=w359:dbl)  [unwired: 2 out]
                n198 = Unbundle(w342) -> ("1 (TL) cal"=w358:dbl, "1 (TN) cal"=w357:dbl, "2 (TL) cal"=w356:dbl, "2 (TN) cal"=w355:dbl)  [unwired: 8 out]
                n199 = local read "LAB05 (SIGNALS)"() -> (w354:T3)
                n200 = Multiply(x=w362, y=w358) -> (x*y=w346:dbl)
                n201 = Multiply(x=w361, y=w357) -> (x*y=w345:dbl)
                n202 = Multiply(x=w360, y=w356) -> (x*y=w343:dbl)
                n203 = Multiply(x=w359, y=w355) -> (x*y=w344:dbl)
                n204 = Bundle By Name(cluster=w354, "1 (TL)"=w346, "1 (TN)"=w345, "2 (TL)"=w343, "2 (TN)"=w344) -> (w353:T3)
                n205 = local write "LAB05 (SIGNALS)"(w353) -> ()
                n206 = Multiply(x=w344, y=w347) -> (x*y=→"5-2(TN) Run":dbl)
                n207 = Multiply(x=w343, y=w347) -> (x*y=→"5-2(TL) Run":dbl)
                n208 = Multiply(x=w345, y=w347) -> (x*y=→"5-1(TN) Run":dbl)
                n209 = Multiply(x=w346, y=w347) -> (x*y=→"5-1(TL) Run":dbl)
              }
            }
          }
        }
      }
    }
    frame #3 {
      # "save all calibration data"
      n210 = String To Path(string=w365) -> (path=w364:path)
      n211 = call <userlib>:"Create Dir if Non-Existant__ogtk.vi"("Directory Path"=w364) -> ("dup Directory Path"=w363:path)  [unwired: 8 in, 2 out]
      n212 = stacked-sequence {
        tunnel: w365 -> [w380 w391 w402 w413 w424 w435]
        tunnel: w370 -> [w379 _ _ _ _ _]
        tunnel: w369 -> [_ w382 _ _ _ _]
        tunnel: w368 -> [_ _ w393 _ _ _]
        tunnel: w367 -> [_ _ _ w404 _ _]
        tunnel: w366 -> [_ _ _ _ w416 _]
        tunnel: w363 -> [_ _ _ _ _ _]
        frame #0 {
          # "LAB01"
          n213 = Concatenate Strings(w380, w379) -> (w381:string)
          n214 = String To Path(string=w381) -> (path=w378:path)
          n215 = Open/Create/Replace File(file path (use dialog)=w378, operation (0:open)=T6."replace or create") -> (refnum out=w377:refnum<file>, error out=w376:errorcluster)  [unwired: 4 in, 1 out]
          n216 = local read "LAB01 (CAL)"() -> (w372:T2)
          n217 = Write to Binary File(file (use dialog)=w377, data=w372, error in=w376) -> (refnum out=w375:refnum<file>, error out=w374:errorcluster)  [unwired: 3 in, 1 out]
          n218 = Close File(refnum=w375, error in=w374) -> (error out=w373:errorcluster)  [unwired: 1 out]
          n219 = local write "file error out"(w373) -> ()
        }
        frame #1 {
          # "LAB02"
          n220 = Concatenate Strings(w391, w382) -> (w392:string)
          n221 = String To Path(string=w392) -> (path=w390:path)
          n222 = Open/Create/Replace File(file path (use dialog)=w390, operation (0:open)=4) -> (refnum out=w389:refnum<file>, error out=w388:errorcluster)  [unwired: 4 in, 1 out]
          n223 = local read "LAB02 (CAL)"() -> (w383:T4)
          n224 = Write to Binary File(file (use dialog)=w389, data=w383, error in=w388) -> (refnum out=w387:refnum<file>, error out=w386:errorcluster)  [unwired: 3 in, 1 out]
          n225 = Close File(refnum=w387, error in=w386) -> (error out=w385:errorcluster)  [unwired: 1 out]
          n226 = local write "file error out"(w385) -> ()
        }
        frame #2 {
          # "LAB03"
          n227 = Concatenate Strings(w402, w393) -> (w403:string)
          n228 = String To Path(string=w403) -> (path=w401:path)
          n229 = Open/Create/Replace File(file path (use dialog)=w401, operation (0:open)=4) -> (refnum out=w400:refnum<file>, error out=w399:errorcluster)  [unwired: 4 in, 1 out]
          n230 = local read "LAB03 (CAL)"() -> (w394:T2)
          n231 = Write to Binary File(file (use dialog)=w400, data=w394, error in=w399) -> (refnum out=w398:refnum<file>, error out=w397:errorcluster)  [unwired: 3 in, 1 out]
          n232 = Close File(refnum=w398, error in=w397) -> (error out=w396:errorcluster)  [unwired: 1 out]
          n233 = local write "file error out"(w396) -> ()
        }
        frame #3 {
          # "LAB04"
          n234 = Concatenate Strings(w413, w404) -> (w414:string)
          n235 = String To Path(string=w414) -> (path=w412:path)
          n236 = Open/Create/Replace File(file path (use dialog)=w412, operation (0:open)=4) -> (refnum out=w411:refnum<file>, error out=w410:errorcluster)  [unwired: 4 in, 1 out]
          n237 = local read "LAB04 (CAL)"() -> (w405:T2)
          n238 = Write to Binary File(file (use dialog)=w411, data=w405, error in=w410) -> (refnum out=w409:refnum<file>, error out=w408:errorcluster)  [unwired: 3 in, 1 out]
          n239 = Close File(refnum=w409, error in=w408) -> (error out=w407:errorcluster)  [unwired: 1 out]
          n240 = local write "file error out"(w407) -> ()
        }
        frame #4 {
          # "LAB05"
          n241 = Concatenate Strings(w424, w416) -> (w425:string)
          n242 = String To Path(string=w425) -> (path=w423:path)
          n243 = local read "LAB05 (CAL) 2"() -> (w415:T5)
          n244 = Open/Create/Replace File(file path (use dialog)=w423, operation (0:open)=4) -> (refnum out=w422:refnum<file>, error out=w421:errorcluster)  [unwired: 4 in, 1 out]
          n245 = Write to Binary File(file (use dialog)=w422, data=w415, error in=w421) -> (refnum out=w420:refnum<file>, error out=w419:errorcluster)  [unwired: 3 in, 1 out]
          n246 = Close File(refnum=w420, error in=w419) -> (error out=w418:errorcluster)  [unwired: 1 out]
          n247 = local write "file error out"(w418) -> ()
        }
        frame #5 {
          # "TEMP REF"
          n248 = Concatenate Strings(w435, "T-REF-cal.bin") -> (w436:string)
          n249 = String To Path(string=w436) -> (path=w434:path)
          n250 = Open/Create/Replace File(file path (use dialog)=w434, operation (0:open)=4) -> (refnum out=w433:refnum<file>, error out=w432:errorcluster)  [unwired: 4 in, 1 out]
          n251 = local read "TEMP REF cal"() -> (w427:dbl)
          n252 = Write to Binary File(file (use dialog)=w433, data=w427, error in=w432) -> (refnum out=w431:refnum<file>, error out=w430:errorcluster)  [unwired: 3 in, 1 out]
          n253 = Close File(refnum=w431, error in=w430) -> (error out=w429:errorcluster)  [unwired: 1 out]
          n254 = local write "file error out"(w429) -> ()
        }
      }
    }
  }
